vi "CloseDISession.vi"(8 "error in (no error)":errorcluster, 10 "gRPCid":T5, 11 "DIOSessions In":T1={"Array of DI Sessions"=[], "Array of DO Sessions"=[], "Stream ReadDI"={"gRPCid ReadDI"=0, "DISessionName"="", "Stream Status ReadDI"=FALSE, "Async Stop ReadDI Queue"=refnum, "DI Task"="", "ms to wait"=500}}) -> (0 "error out":errorcluster, 3 "DIOSessions Out":T1={"Array of DI Sessions"=[], "Array of DO Sessions"=[], "Stream ReadDI"={"gRPCid ReadDI"=0, "DISessionName"="", "Stream Status ReadDI"=FALSE, "Async Stop ReadDI Queue"=refnum, "DI Task"="", "ms to wait"=500}})   [LabVIEW 2019, in "ctet_dio_User Library.lvlib"]
uses:
  ctet_dio_User Library.lvlib
  Servers/ctet_dio/gRPC lvSupport/Server API/typeDefs/grpcId.ctl
  Types/DIOSessions.ctl
  Types/DISession.ctl
  Types/DOSession.ctl
  Types/StreamReadDI.ctl
  Servers/ctet_dio/ctet_dio Class/RPC Messages/measurementservice_DICloseSessionResponse/measurementservice_DICloseSessionResponse_Data.ctl
  Servers/ctet_dio/ctet_dio Class/RPC Messages/measurementservice_ErrorOut/measurementservice_ErrorOut_Data.ctl
  Servers/ctet_dio/ctet_dio Class/ctet_dio.lvclass
  Servers/ctet_dio/gRPC lvSupport/gprc-lvsupport.lvlib
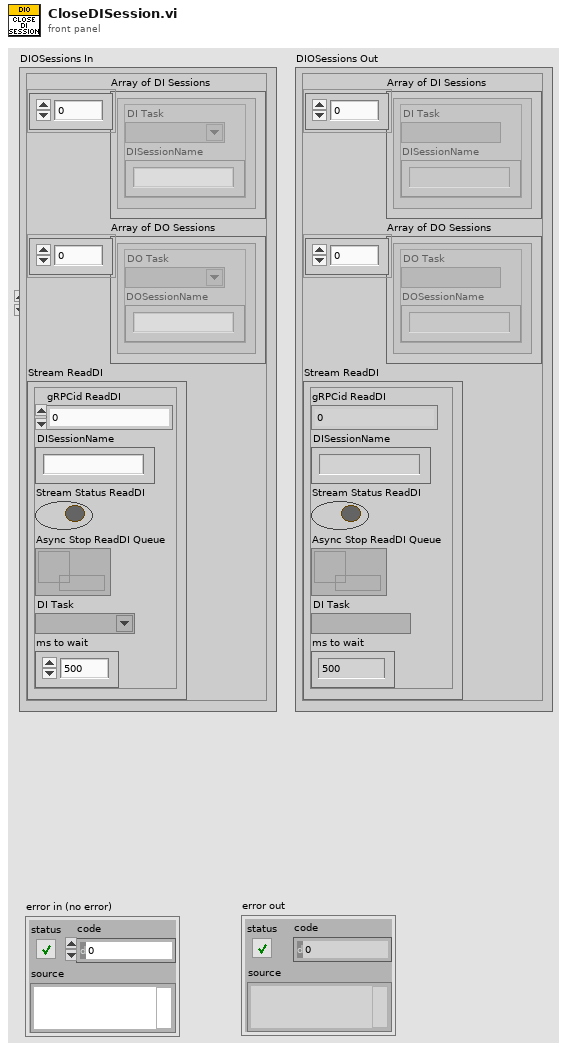
[diagram p1: front panel]
types:
  T1 = typedef "ctet_dio_User Library.lvlib/DIOSessions.ctl" = cluster{"Array of DI Sessions":T2[], "Array of DO Sessions":T3[], "Stream ReadDI":T4}
  T2 = typedef "ctet_dio_User Library.lvlib/DISession.ctl" = cluster{"DI Task":refnum<k21>, "DISessionName":string}
  T3 = typedef "ctet_dio_User Library.lvlib/DOSession.ctl" = cluster{"DO Task":refnum<k21>, "DOSessionName":string}
  T4 = typedef "ctet_dio_User Library.lvlib/StreamReadDI.ctl" = cluster{"gRPCid ReadDI":T5, "DISessionName":string, "Stream Status ReadDI":bool, "Async Stop ReadDI Queue":refnum<queue>, "DI Task":refnum<k21>, "ms to wait":u32}
  T5 = typedef "ctet_dio.lvlib/gprc-lvsupport.lvlib/grpcId.ctl" = u64
  T6 = typedef "ctet_dio.lvlib/ctet_dio.lvclass/measurementservice_ErrorOut_Data.ctl" = cluster{"errCode":i64, "errMessage":string}
  T7 = typedef "ctet_dio.lvlib/ctet_dio.lvclass/measurementservice_DICloseSessionResponse_Data.ctl" = cluster{"error":T6}
  T8 = typedef "ctet_dio.lvlib/ctet_dio.lvclass/measurementservice_DICloseSessionRequest_Data.ctl" = cluster{"DISessionName":string}
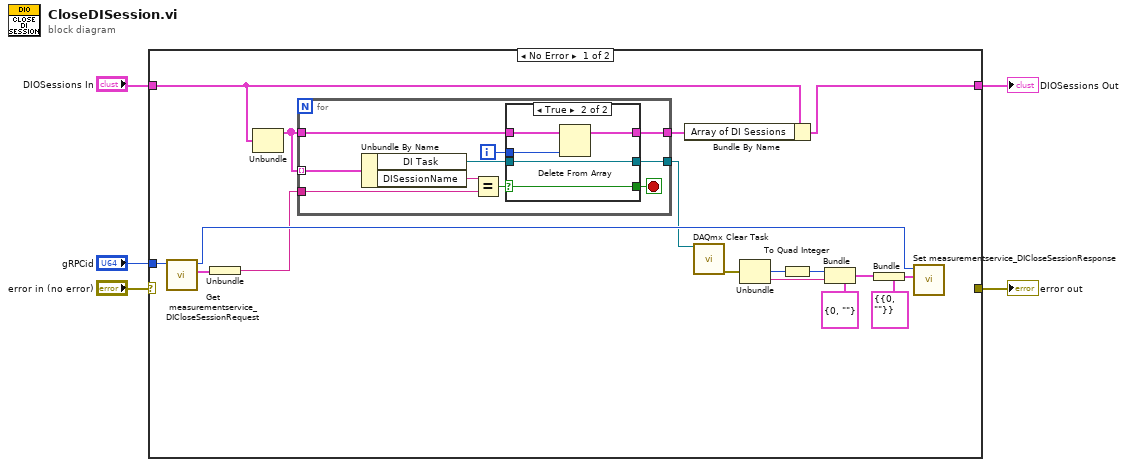
[diagram p0: block diagram]
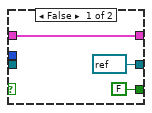
[diagram p2: hidden frame]
diagram:
  n1 = case shown="No Error" "error in (no error)" {
    selector: "error in (no error)" -> [_ w42]
    tunnel: [_ w42] -> w5
    tunnel: "gRPCid" -> [w22 _]
    tunnel: "DIOSessions In" -> [w11 w41]
    tunnel: [w10 w41] -> w1
    frame No Error {
      n2 = call "Get measurementservice_DICloseSessionRequest.vi"("gRPCid"=w22) -> ("Message Data"=w21:T8, "gRPCid out"=w18:T5)  [unwired: 8 in, 1 out]
      n3 = Unbundle(w21) -> ("DISessionName"=w9:string)
      n4 = Unbundle(w11) -> ("Array of DI Sessions"=w13:T2[])  [unwired: 2 out]
      n5 = for {
        tunnel: w13 -> [w27] mode=indexing
        tunnel: w9 -> [w32]
        tunnel: [w28] -> w14
        tunnel: w13 -> [w26]
        tunnel: [w25] -> w12
        i -> [w23]
        stop <- w30 stop-if-true
        n6 = Unbundle By Name(w27) -> ("DI Task"=w29:refnum<k21>, "DISessionName"=w24:string)
        n7 = Equal?(x=w24, y=w32) -> (x = y?=w31:bool)
        n8 = case shown="True" w31 {
          selector: w31 -> [_ w40]
          tunnel: [FALSE w40] -> w30
          tunnel: w29 -> [_ w38]
          tunnel: [refnum<k21> refnum ("DI Task") w38] -> w28
          tunnel: w26 -> [w33 w39]
          tunnel: [w33 w36] -> w25
          tunnel: w23 -> [_ w37]
          frame False {
          }
          frame True {
            n9 = Delete From Array(array=w39, index=w37) -> (array with subset deleted=w36:T2[])  [unwired: 1 in, 1 out]
          }
        }
      }
      n10 = Bundle By Name(cluster=w11, "Array of DI Sessions"=w12) -> (w10:T1)
      n11 = call <vilib>:"DAQmx Clear Task.vi"("task in"=w14) -> ("error out"=w15:errorcluster)  [unwired: 14 in]
      n12 = Unbundle(w15) -> ("code"=w7:i32, "source"=w8:string)  [unwired: 1 out]
      n13 = To Quad Integer(1:w7) -> (0:w6:i64)
      n14 = Bundle(cluster=T6 {"errCode"=0, "errMessage"=""} ("error"), "errCode"=w6, "errMessage"=w8) -> (w16:T6)
      n15 = Bundle(cluster=T7 {"error"={"errCode"=0, "errMessage"=""}} ("measurementservice_DICloseSessionResponse_Data"), "error"=w16) -> (w19:T7)
      n16 = call "Set measurementservice_DICloseSessionResponse.vi"("Message Data"=w19, "gRPCid"=w18) -> ()  [unwired: 9 in, 1 out]
    }
    frame Error {
    }
  }
  "error out" <- w5
  "DIOSessions Out" <- w1
